vi "Cell Space_ListBox.vi"(4 "Row Header in":string[](array[string]), 6 "Col Header in":string[](array[string]), 7 "빈내용 숨기기?(F)":bool, 8 "error in":errorcluster caption="에러 입력(에러 없음)", 10 "Data in":string[][](array[string]), 11 "여러열리스트박스 참조 in":refnum<vi>) -> (0 "error out":errorcluster caption="에러 출력", 3 "여러열리스트박스 참조 out":refnum<vi>)   [LabVIEW 2020]
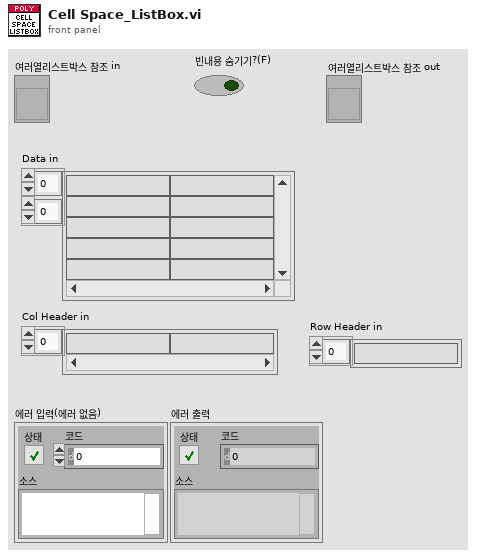
[diagram p1: front panel]
types:
  T1 = cluster{"left":i16, "top":i16, "right":i16, "bottom":i16}
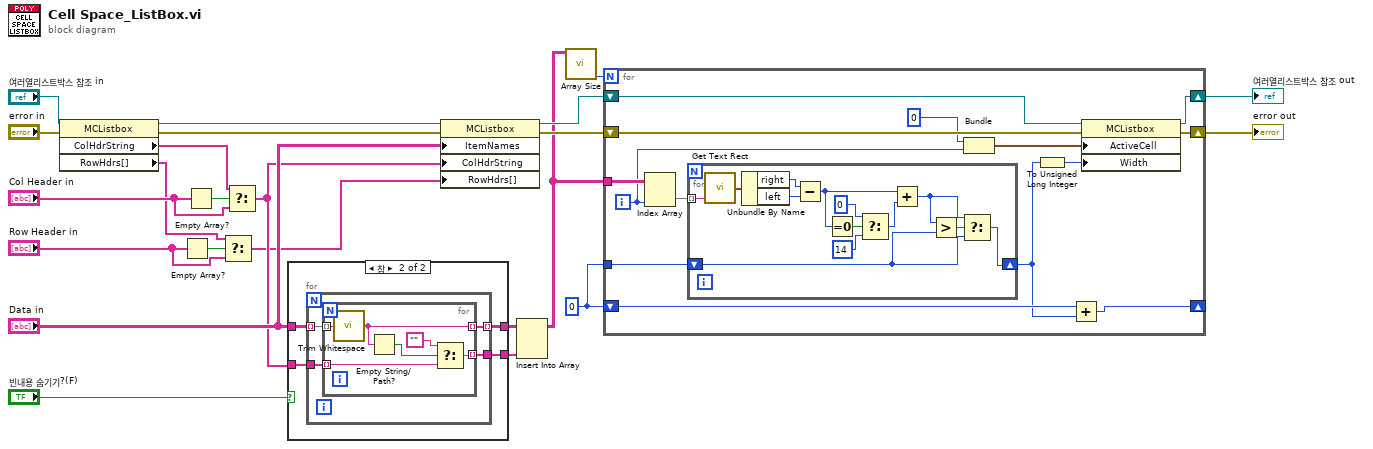
[diagram p0: block diagram]
diagram:
  w21 = i16 0 ("인덱스")
  n1 = property on="프로퍼티 노드" class="MCListbox"(reference="여러열리스트박스 참조 in", error in="error in") -> (reference out=w11:refnum<vi>, error out=w12:errorcluster, "ColHdrString"=w9:string[], "RowHdrs[]"=w5:string[])
  n2 = Empty Array?(array="Row Header in") -> (empty?=w6:bool)
  n3 = Empty Array?(array="Col Header in") -> (empty?=w10:bool)
  n4 = Select(t=w5, s=w6, f="Row Header in") -> (s? t:f=w3:string[])
  n5 = Select(t=w9, s=w10, f="Col Header in") -> (s? t:f=w7:string[])
  n6 = case shown="참" "빈내용 숨기기?(F)" {
    tunnel: "Data in" -> [w25 w29]
    tunnel: [w25 w28] -> w20
    tunnel: w7 -> [w24 w27]
    tunnel: [w24 w26] -> w19
    frame False {
    }
    frame True {
      n7 = for {
        tunnel: w29 -> [w33] mode=indexing
        tunnel: [w32] -> w28 mode=indexing
        tunnel: w27 -> [w31]
        tunnel: [w30] -> w26
        n8 = for {
          tunnel: w33 -> [w39] mode=indexing
          tunnel: [w38] -> w32 mode=indexing
          tunnel: w31 -> [w36] mode=indexing
          tunnel: [w35] -> w30 mode=indexing
          n9 = call <vilib>:"Trim Whitespace.vi"("string"=w39) -> ("trimmed string"=w38:string)  [unwired: 1 in]
          n10 = Empty String/Path?(string/path=w38) -> (empty?=w37:bool)
          n11 = Select(t="", s=w37, f=w36) -> (s? t:f=w35:string)
        }
      }
    }
  }
  n12 = property on="프로퍼티 노드" class="MCListbox"(reference=w11, error in=w12, "ItemNames"="Data in", "ColHdrString"=w7, "RowHdrs[]"=w3) -> (reference out=w15:refnum<vi>, error out=w17:errorcluster)
  n13 = Insert Into Array(array=w20, new element=w19) -> (w2:string[][])  [unwired: 2 in]
  n14 = call "Array Size.vi"("Data in"=w2) -> ("열(I32)"=w1:i32)  [unwired: 7 in, 3 out]
  n15 = for {
    N: w1 -> [_]
    shift-right: [w52] -> w23
    shift-left: w17 -> [w53]
    tunnel: w2 -> [w51]
    shift-right: [w45] -> _
    shift-left: w21 -> [w44]
    shift-right: [w42] -> w22
    shift-left: w15 -> [w46]
    tunnel: w21 -> [w41]
    i -> [w49]
    n16 = Index Array(array=w51, index (col)=w49) -> (element=w50:string[])  [unwired: 1 in]
    n17 = for {
      tunnel: w50 -> [w63] mode=indexing
      shift-right: [w64] -> w43
      shift-left: w41 -> [w65]
      n18 = call <vilib>:"Get Text Rect.vi"("text"=w63) -> ("rect"=w62:T1)  [unwired: 8 in]
      n19 = Unbundle By Name(w62) -> ("right"=w61:i16, "left"=w60:i16)
      n20 = Subtract(x=w61, y=w60) -> (x-y=w58:i16)
      n21 = Equal To 0?(x=w58) -> (x = 0?=w57:bool)
      n22 = Select(t=i16 0 ("y"), s=w57, f=i16 14 ("y")) -> (s? t:f=w54:i16)
      n23 = Add(x=w58, y=w54) -> (x+y=w59:i16)
      n24 = Greater?(x=w59, y=w65) -> (0:w66:bool)
      n25 = Select(t=w59, s=w66, f=w65) -> (s? t:f=w64:i16)
    }
    n26 = Bundle("인덱스"=0, w49) -> (w47:cluster{"인덱스":i32, i32})  [unwired: 1 in]
    n27 = To Unsigned Long Integer(number=w43) -> (unsigned 32bit integer=w40:u32)
    n28 = Add(x=w44, y=w43) -> (x+y=w45:i16)
    n29 = property on="프로퍼티 노드" class="MCListbox"(reference=w46, error in=w53, "ActiveCell"=w47, "Width"=w40) -> (reference out=w42:refnum<vi>, error out=w52:errorcluster)
  }
  "error out" <- w23
  "여러열리스트박스 참조 out" <- w22
